vi "TEST Array Operation.vi"() -> ()   [LabVIEW 2013, in "Carya Config.lvclass"]
doc: "Copyright 2018, Carya Automatisering, Wiebe Walstra."
uses:
  Carya Config.lvclass
panel:
  in  "String 3":string="\n[one]\nkey=this is only a test\n\n[two]\nkey=this is only a test\narray0=0,1,2,3,4,5,6,7,8,9\narray1=\narray2="
  out "String":string
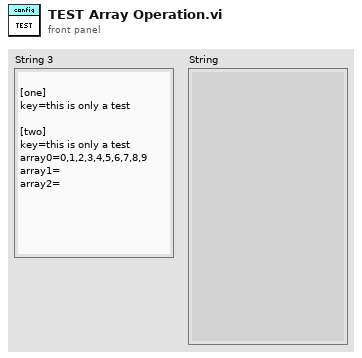
[diagram p1: front panel]
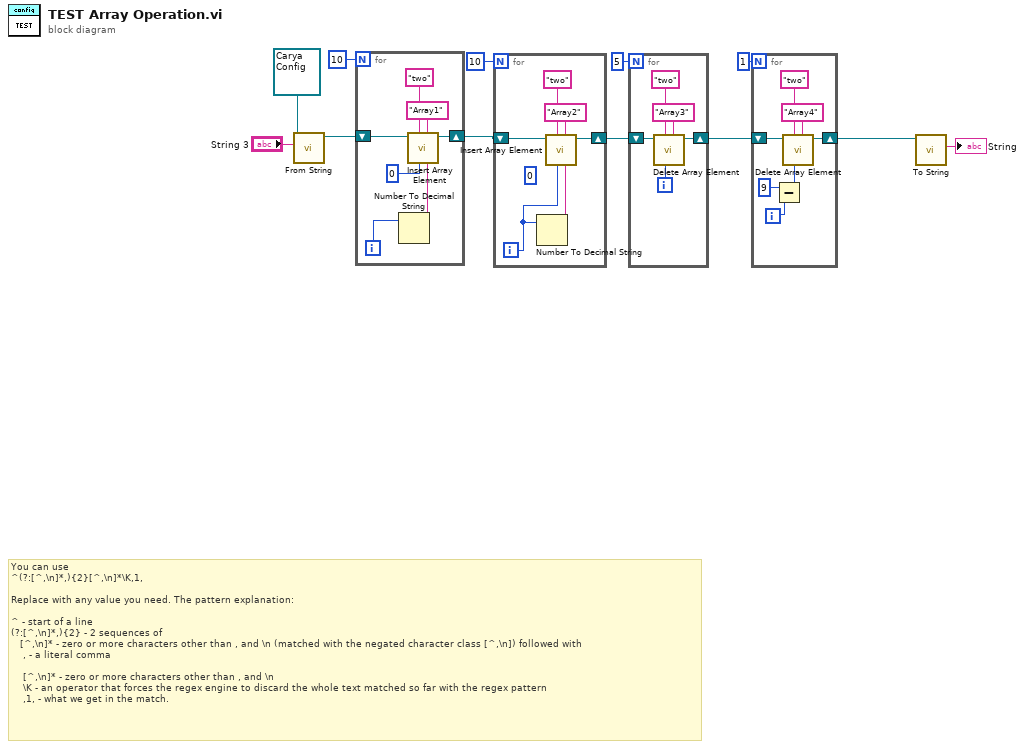
[diagram p0: block diagram]
diagram:
  # "You can use\n^(?:[^,\\n]*,){2}[^,\\n]*\\K,1,\n\nReplace with any value you need. The pattern explanation:\n\n^ - start of a line\n(?:[^,\\n]*,){2} - 2 sequences of \n   [^,\\n]* - zero or more characters other than , and \\n (matched with the negated character class [^,\\n]) followed with\n    , - a literal comma\n\n    [^,\\n]* - zero or more characters other than , and \\n \n    \\K - an operator that forces the regex engine to discard the whole text matched so far with the regex pattern\n    ,1, - what we get in the match."
  n1 = call-dynamic "From String.vi"("String"="String 3", "Carya Config in"=refnum<class "Carya Config.lvclass"> refnum) -> ("Carya Config out"=w9:refnum<class "Carya Config.lvclass">)  [unwired: 7 in, 2 out]
  n2 = for {
    N: 10 -> [_]
    shift-right: [w15] -> w7
    shift-left: w9 -> [w19]
    i -> [w14]
    n3 = Number To Decimal String(number=w14) -> (decimal integer string=w13:string)  [unwired: 1 in]
    n4 = call-dynamic "Insert Array Element.vi"("Insert"=w13, "Key name"="Array1", "Index"=0, "Section name"="two", "Carya Config in"=w19) -> ("Carya Config out"=w15:refnum<class "Carya Config.lvclass">)  [unwired: 5 in, 1 out]
  }
  n5 = for {
    N: 10 -> [_]
    shift-right: [w22] -> w5
    shift-left: w7 -> [w25]
    i -> [w20]
    (unwired) 0 ("Index")
    n6 = Number To Decimal String(number=w20) -> (decimal integer string=w21:string)  [unwired: 1 in]
    n7 = call-dynamic "Insert Array Element.vi"("Insert"=w21, "Key name"="Array2", "Index"=w20, "Section name"="two", "Carya Config in"=w25) -> ("Carya Config out"=w22:refnum<class "Carya Config.lvclass">)  [unwired: 5 in, 1 out]
  }
  n8 = for {
    N: 5 -> [_]
    shift-right: [w27] -> w2
    shift-left: w5 -> [w30]
    i -> [w26]
    n9 = call-dynamic "Delete Array Element.vi"("Key name"="Array3", "Index"=w26, "Section name"="two", "Carya Config in"=w30) -> ("Carya Config out"=w27:refnum<class "Carya Config.lvclass">)  [unwired: 6 in, 1 out]
  }
  n10 = for {
    N: 1 -> [_]
    shift-right: [w34] -> w1
    shift-left: w2 -> [w37]
    i -> [w31]
    n11 = Subtract(x=9, y=w31) -> (x-y=w33:i32)
    n12 = call-dynamic "Delete Array Element.vi"("Key name"="Array4", "Index"=w33, "Section name"="two", "Carya Config in"=w37) -> ("Carya Config out"=w34:refnum<class "Carya Config.lvclass">)  [unwired: 6 in, 1 out]
  }
  n13 = call-dynamic "To String.vi"("Carya Config in"=w1) -> ("String"=→"String":string)  [unwired: 8 in, 2 out]
